vi "Unit Test Preserve wired non-serialized data (Same) False.vi"() -> ()   [LabVIEW 2019, in "Sports Unit Tests.lvclass"]
uses:
  Sports Unit Tests.lvclass
  <vilib>/addons/_JKI Toolkits/Caraya/classes/Assert/Assert.lvclass
  Classes/Adam Sandler/Adam Sandler.lvclass
  <vilib>/addons/_JKI Toolkits/Caraya/classes/Assert/Assert Equal Value_Variant.vi
  <vilib>/addons/_JKI Toolkits/Caraya/classes/Assert/Assert Not Error.vi
  <userlib>/Blue Origin/BlueSerialization/BlueSerializer/DeserializeMutationOptions.ctl
  <userlib>/Blue Origin/BlueSerialization/BlueSerializer/BlueSerializer.lvclass
  <userlib>/Blue Origin/BlueSerialization/BlueSerializer/DeserializeSlicingOptions.ctl
  <userlib>/Blue Origin/BlueSerialization/BlueSerializer/DeserializeOptions.ctl
  <userlib>/Blue Origin/BlueSerialization/BlueSerializer/DeserializePreservationOptions.ctl
  <userlib>/Blue Origin/BlueSerialization/BlueSerializer/PreserveNonWiredDataOption.ctl
panel:
  out "Table":string[][](table)
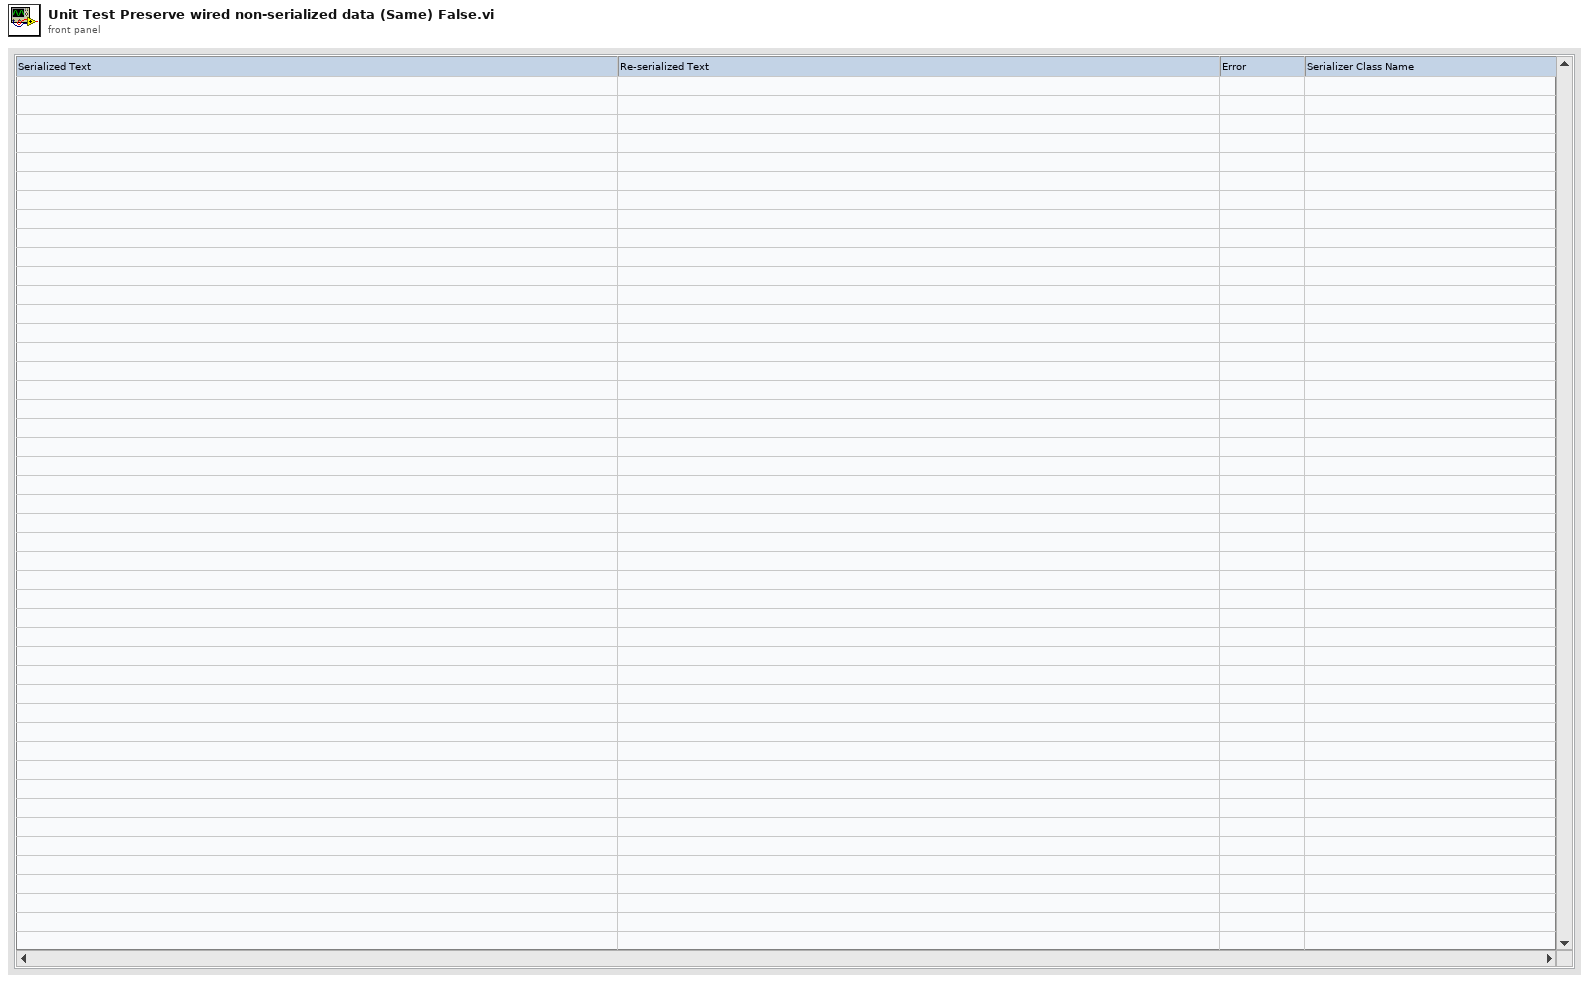
[diagram p1: front panel]
types:
  T1 = typedef "BlueSerialization.lvlib/BlueSerializer.lvclass/PreserveNonWiredDataOption.ctl" = enum16{"Don't preserve", "Preserve (error on less-specific wired types)", "Preserve (except on less-specific wired types)"}
  T2 = typedef "BlueSerialization.lvlib/BlueSerializer.lvclass/DeserializeOptions.ctl" = cluster{"deserialize non-BlueSerializable objects from hex?":bool, "expand objects on type conflict?":bool, "Slicing":T3, "Mutation Options":T4, "Preservation Options":T5}
  T3 = typedef "BlueSerialization.lvlib/BlueSerializer.lvclass/DeserializeSlicingOptions.ctl" = cluster{"slice flattened object data on error?":bool, "sliceable class names":string[]}
  T4 = typedef "BlueSerialization.lvlib/BlueSerializer.lvclass/DeserializeMutationOptions.ctl" = cluster{"error on inserted parent levels?":bool, "\terror on obsolete parent levels?":bool}
  T5 = typedef "BlueSerialization.lvlib/BlueSerializer.lvclass/DeserializePreservationOptions.ctl" = cluster{"Preserve wired serialized data?":bool, "Preserve wired non-serialized data":T1}
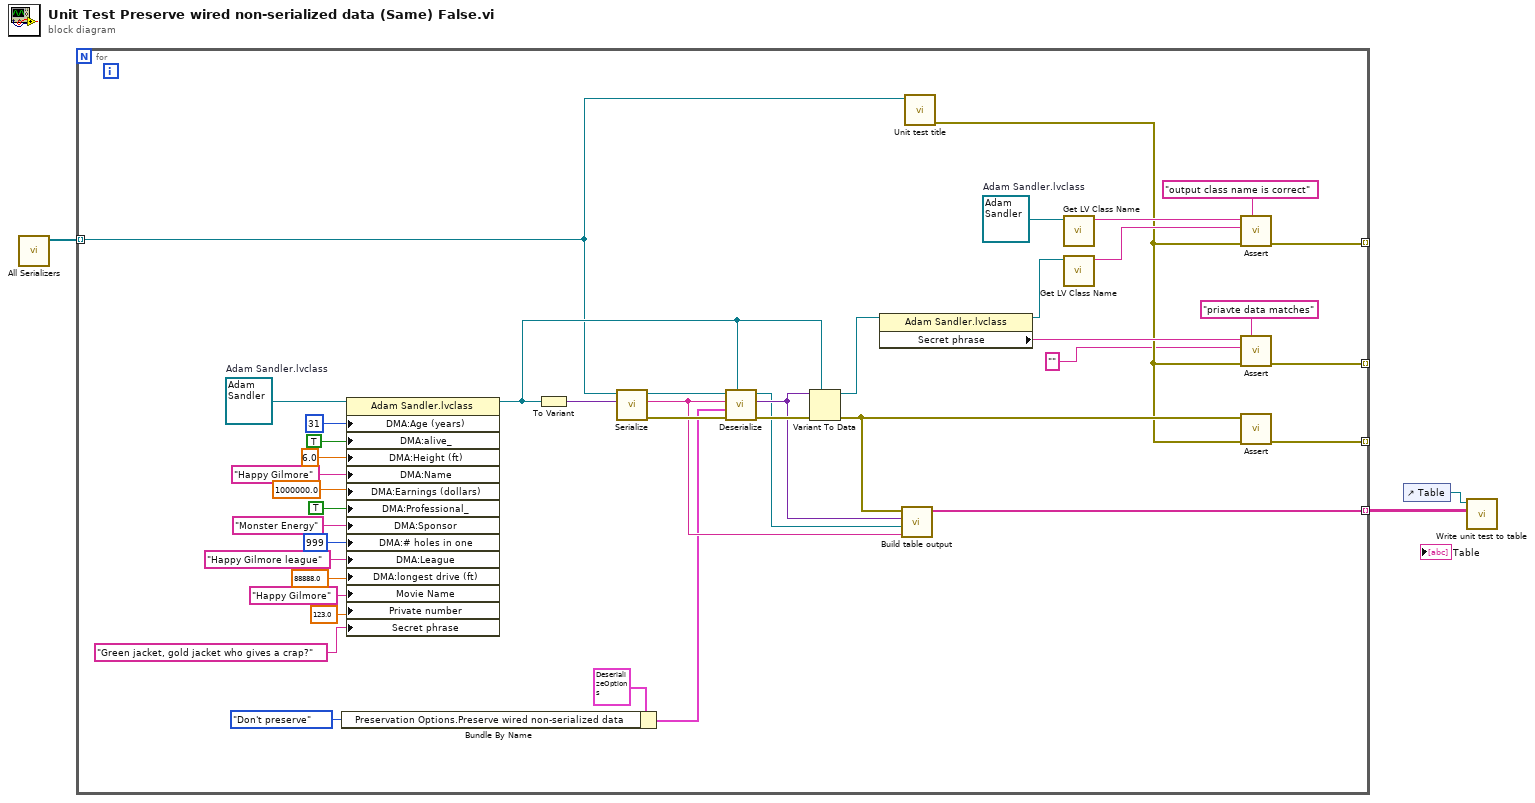
[diagram p0: block diagram]
diagram:
  n1 = call "All Serializers.vi"() -> ("All serializers"=w2:refnum<class "BlueSerializer.lvclass">[])  [unwired: 11 in]
  n2 = for {
    tunnel: w2 -> [w5] mode=indexing
    tunnel: [w30] -> _ mode=indexing
    tunnel: [w29] -> _ mode=indexing
    tunnel: [w24] -> w1 mode=indexing
    tunnel: [w10] -> _ mode=indexing
    w17 = refnum<class "Adam Sandler.lvclass"> refnum  # Adam Sandler.lvclass
    w23 = refnum<class "Adam Sandler.lvclass"> refnum  # Adam Sandler.lvclass
    n3 = Bundle By Name(cluster=T2 {"deserialize non-BlueSerializable objects from hex?"=FALSE, "expand objects on type conflict?"=FALSE, "Slicing"={"slice flattened object data on error?"=FALSE, "sliceable class names"=[]}, "Mutation Options"={"error on inserted parent levels?"=FALSE, "\terror on obsolete parent levels?"=FALSE}, "Preservation Options"={"Preserve wired serialized data?"=FALSE, "Preserve wired non-serialized data"=enum."Don't preserve"}} ("Deserialize Options"), "Preservation Options.Preserve wired non-serialized data"=PreserveNonWiredDataOption."Don't preserve") -> (w6:T2)
    n4 = property on="Property Node" class="Adam Sandler.lvclass"(reference=w23, "DMA:Age (years)"=u16 31 ("Age (years)"), "DMA:alive_"=TRUE ("alive_"), "DMA:Height (ft)"=6.0 ("Height (ft)"), "DMA:Name"="Happy Gilmore" ("Name"), "DMA:Earnings (dollars)"=1000000.0 ("Earnings (dollars)"), "DMA:Professional_"=TRUE ("Professional_"), "DMA:Sponsor"="Monster Energy" ("Sponsor"), "DMA:# holes in one"=999 ("# holes in one"), "DMA:League"="Happy Gilmore league" ("League"), "DMA:longest drive (ft)"=88888.0 ("longest drive (ft)"), "Movie Name"="Happy Gilmore", "Private number"=123.0, "Secret phrase"="Green jacket, gold jacket who gives a crap?") -> (reference out=w9:refnum<class "Adam Sandler.lvclass">)  [unwired: 1 in, 1 out]
    n5 = To Variant(anything=w9) -> (Variant=w42:variant)
    n6 = call <userlib>:"Serialize.vi"("Anything"=w42, "BlueSerializer in"=w5) -> ("error out"=w44:errorcluster, "Serialized Text"=w25:string, "BlueSerializer out"=w43:refnum<class "BlueSerializer.lvclass">)  [unwired: 7 in]
    n7 = call <userlib>:"Deserialize.vi"("Anything"=w9, "error in (no error)"=w44, "Deserialize Options"=w6, "Serialized Text"=w25, "BlueSerializer in"=w43) -> ("error out"=w41:errorcluster, "Variant"=w27:variant, "BlueSerializer out"=w26:refnum<class "BlueSerializer.lvclass">)  [unwired: 4 in]
    n8 = Variant To Data(error in=w41, type=w9, Variant=w27) -> (data=w15:refnum<class "Adam Sandler.lvclass">, error out=w28:errorcluster)
    n9 = property class="Adam Sandler.lvclass"(reference=w15) -> (reference out=w14:refnum<class "Adam Sandler.lvclass">, "Secret phrase"=w13:string)  [unwired: 1 in, 1 out]
    n10 = call "Build table output.vi"("serialized text"=w25, "BlueSerializer in"=w26, "deserialized variant"=w27, "variant to data error"=w28) -> ("table output"=w24:string[])  [unwired: 7 in]
    n11 = call "Unit test title.vi"("serializer"=w5) -> ("error out"=w11:errorcluster)  [unwired: 9 in, 1 out]
    n12 = call <vilib>:"Get LV Class Name.vi"("object"=w17) -> ("class name"=w40:string)  [unwired: 9 in, 1 out]
    n13 = call <vilib>:"Get LV Class Name.vi"("object"=w14) -> ("class name"=w39:string)  [unwired: 9 in, 1 out]
    n14 = call-poly <vilib>:"Assert.vi"("Label"="output class name is correct", "error in (no error)"=w11, "Y"=w39, "X"=w40) -> ("error out"=w29:errorcluster)  [unwired: 7 in]
    n15 = call-poly <vilib>:"Assert.vi"("Label"="priavte data matches", "error in (no error)"=w11, "Y"="" ("Secret phrase"), "X"=w13) -> ("error out"=w10:errorcluster)  [unwired: 7 in]
    n16 = call-poly <vilib>:"Assert.vi"("error in (no error)"=w11, "Not Error?"=w28) -> ("error out"=w30:errorcluster)  [unwired: 9 in]
  }
  n17 = control-ref of="Table"() -> (w3:refnum<vi>)
  n18 = call "Write unit test to table.vi"("Table"=w1, "Table ref in"=w3) -> ()  [unwired: 9 in, 1 out]
